vi "Query Trace Data.vi"(8 "error in (no error)":errorcluster, 10 "Trace Number":u8=1, 11 "VNA-FieldFox in":refnum<class "VNA-FieldFox.lvclass">) -> (0 "error out":errorcluster, 1 "Data":dbl[](array[numeric]), 2 "Frequency":dbl[](array[numeric]), 3 "VNA-FieldFox out":refnum<class "VNA-FieldFox.lvclass">)   [LabVIEW 2020, in "VNA-FieldFox.lvclass"]
doc: "Query the active trace data.\nIt returns both x and y data"
uses:
  VNA-FieldFox.lvclass
  C:/Sandbox/Git_Sandbox/WiSpry Test Framework source code (LV20)/WiSpry Test Framework/Instruments/Instrument.lvclass
  Instrument.lvclass/Instrument.ctl
  <instrlib>/Agilent N99XX Series/Agilent N99XX Series.lvlib
  Instrument.lvclass
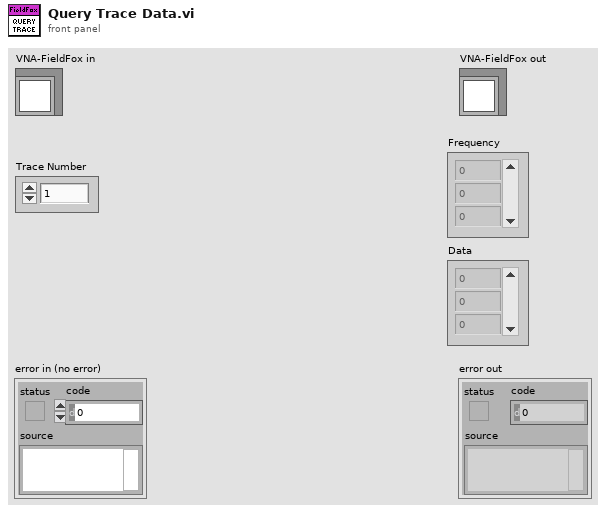
[diagram p1: front panel]
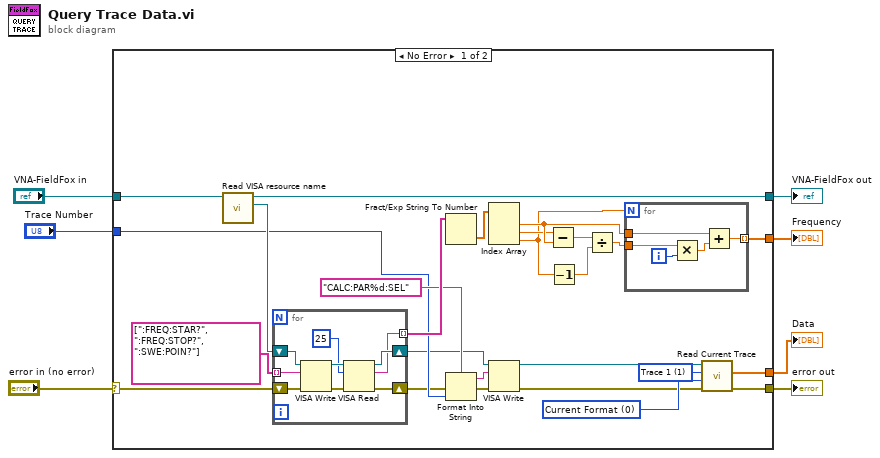
[diagram p0: block diagram]
diagram:
  n1 = case shown="No Error" "error in (no error)" {
    selector: "error in (no error)" -> [w20 w48]
    tunnel: [w33 w48] -> w6
    tunnel: "Trace Number" -> [w15 _]
    tunnel: "VNA-FieldFox in" -> [w32 w49]
    tunnel: [w31 w49] -> w3
    tunnel: [w30 _] -> w2
    tunnel: [w18 _] -> w1
    frame No Error {
      w8 = 1 items=["Trace 1"=1, "Trace 2"=2, "Trace 3"=3, "Trace 4"=4] ("Trace Index (1: Trace 1)")
      w17 = 0 items=["Current Format", "Raw Data"] ("Data Type (0: Current Format)")
      n2 = call "Read VISA resource name.vi"("Instrument in"=w32) -> ("VISA resource name"=w19:refnum<visa-resource-name>, "Instrument out"=w31:refnum<class "VNA-FieldFox.lvclass">)  [unwired: 9 in]
      n3 = for {
        tunnel: string[] [":FREQ:STAR?", ":FREQ:STOP?", ":SWE:POIN?"] -> [w42] mode=indexing
        tunnel: [w41] -> w21 mode=indexing
        shift-right: [w45] -> w14
        shift-left: w19 -> [w46]
        shift-right: [w39] -> w11
        shift-left: w20 -> [w40]
        n4 = VISA Write(VISA resource name=w46, write buffer=w42, error in (no error)=w40) -> (VISA resource name out=w47:refnum<visa-resource-name>, error out=w43:errorcluster)  [unwired: 1 out]
        n5 = VISA Read(VISA resource name=w47, byte count=u32 25, error in (no error)=w43) -> (VISA resource name out=w45:refnum<visa-resource-name>, read buffer=w41:string, error out=w39:errorcluster)  [unwired: 1 out]
      }
      n6 = Fract/Exp String To Number(string=w21) -> (number=w22:dbl[])  [unwired: 3 in, 1 out]
      n7 = Format Into String(format string="CALC:PAR%d:SEL", error in=w11, w15) -> (resulting string=w9:string, error out=w10:errorcluster)  [unwired: 1 in]
      n8 = Index Array(array=w22) -> (element #1=w28:dbl, element #2=w27:dbl, element #3=w25:dbl)  [unwired: 3 in]
      n9 = VISA Write(VISA resource name=w14, write buffer=w9, error in (no error)=w10) -> (VISA resource name out=w12:refnum<visa-resource-name>, error out=w13:errorcluster)  [unwired: 1 out]
      n10 = Subtract(x=w27, y=w28) -> (x-y=w26:dbl)
      n11 = Decrement(x=w25) -> (x-1=w24:dbl)
      n12 = Divide(x=w26, y=w24) -> (x/y=w23:dbl)
      n13 = for {
        N: w25 -> [_]
        tunnel: w28 -> [w38]
        tunnel: w23 -> [w36]
        tunnel: [w34] -> w18 mode=indexing
        i -> [w37]
        n14 = Multiply(x=w36, y=w37) -> (x*y=w35:dbl)
        n15 = Add(x=w38, y=w35) -> (x+y=w34:dbl)
      }
      n16 = call <instrlib>:"Read Current Trace.vi"("error in (no error)"=w13, "Data Type (0: Current Format)"=w17, "Trace Index (1: Trace 1)"=w8, "VISA resource name"=w12) -> ("error out"=w33:errorcluster, "Current Trace Data"=w30:dbl[])  [unwired: 3 in, 3 out]
    }
    frame Error {
    }
  }
  "error out" <- w6
  "VNA-FieldFox out" <- w3
  "Data" <- w2
  "Frequency" <- w1
